vi "PH_GUI.set element in cluster GUI object.vi"(1 "Cluster Ref":refnum<vi>, 2 "Cluster index":i32, 3 "Value":variant, 4 "Blinking? (false)":bool, 5 "error in (no error)":errorcluster, 7 "Grayed out? (false)":bool) -> (19 "error out":errorcluster)   [LabVIEW 2014, in "PH_Common.lvlib"]
doc: "Sets value and more for a certain element the referenced cluster GUI object."
uses:
  PH_Common.lvlib
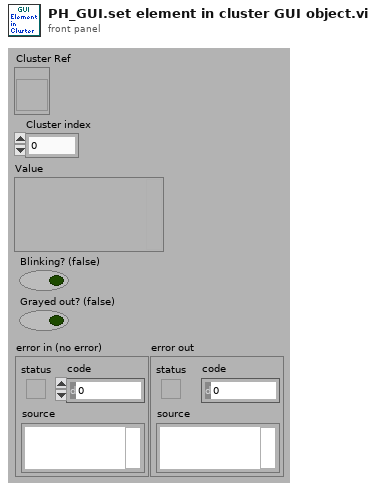
[diagram p1: front panel]
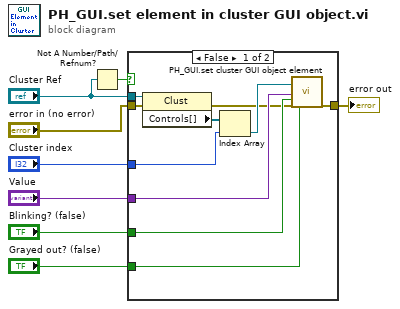
[diagram p0: block diagram]
diagram:
  n1 = Not A Number/Path/Refnum?(number/path/refnum="Cluster Ref") -> (NaN/Path/Refnum?=w3:bool)
  n2 = case shown="False" w3 {
    tunnel: "Cluster index" -> [w18 _]
    tunnel: "error in (no error)" -> [w11 w19]
    tunnel: [w17 w19] -> w6
    tunnel: "Blinking? (false)" -> [w16 _]
    tunnel: "Value" -> [w15 _]
    tunnel: "Cluster Ref" -> [w10 _]
    tunnel: "Grayed out? (false)" -> [w9 _]
    frame False {
      n3 = property class="Clust"(reference=w10, error in=w11) -> (error out=w12:errorcluster, "Controls[]"=w13:refnum<vi>[])  [unwired: 1 out]
      n4 = Index Array(array=w13, index=w18) -> (element=w14:refnum<vi>)
      n5 = call "PH_GUI.set cluster GUI object element.vi"("Ctl Refnum"=w14, "Value"=w15, "Blinking? (false)"=w16, "error in"=w12, "Grayed out? (false)"=w9) -> ("error out"=w17:errorcluster)  [unwired: 14 in]
    }
    frame True {
    }
  }
  "error out" <- w6
